vi "fourier plus standard deviation HASO.vi"(9 "starting frequency bin to plot":i32, 10 "Array in":sgl[][](array[numeric]), 11 "rep rate (Hz)":sgl) -> (1 "Power spectral density":cluster{"f0":dbl, "df":dbl, "magnitude":dbl[]}[](array[cluster]), 2 "Sds":dbl[](array[numeric]), 3 "Power spectra":cluster{"f0":dbl, "df":dbl, "magnitude":dbl[]}[](array[cluster]))   [LabVIEW 2020]
uses:
  <vilib>/Analysis/NI_AALBase.lvlib
panel:
  out "x/y":dbl[](array[numeric])
  out "delta t":sgl
  out "Num points":i32
  out "SDs from Power spectral density":dbl[](array[numeric])
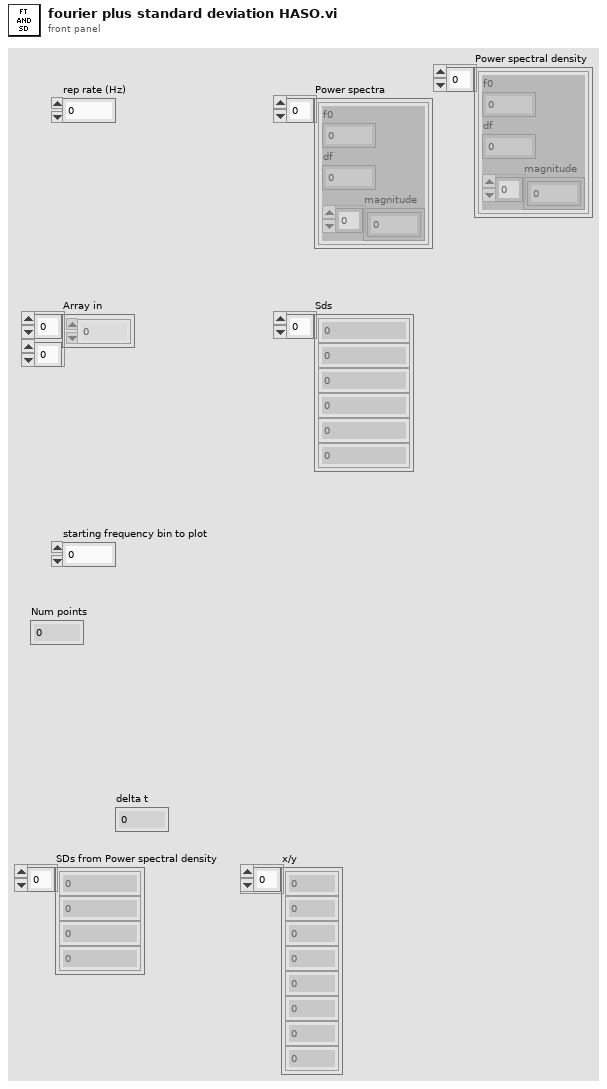
[diagram p1: front panel]
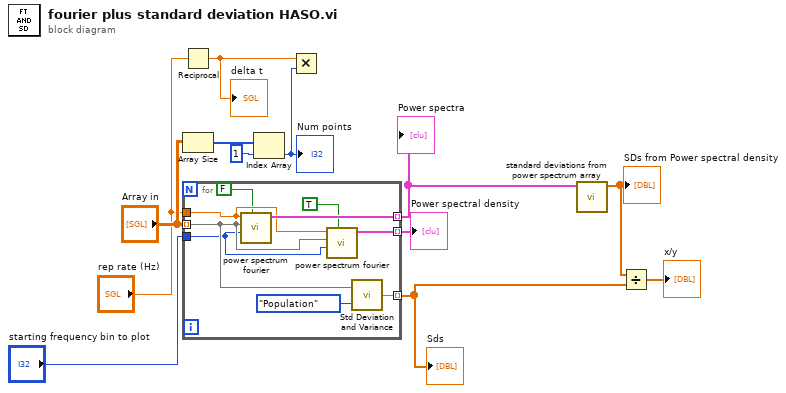
[diagram p0: block diagram]
diagram:
  n1 = Reciprocal(x="rep rate (Hz)") -> (1/x=w6:sgl)
  "delta t" <- w6
  n2 = Array Size(array="Array in") -> (size(s)=w9:i32[])
  n3 = for {
    tunnel: [w21] -> w11 mode=indexing
    tunnel: "starting frequency bin to plot" -> [w15]
    tunnel: "rep rate (Hz)" -> [w17]
    tunnel: "Array in" -> [w16] mode=indexing
    tunnel: [w20] -> w4 mode=indexing
    tunnel: [w14] -> w1 mode=indexing
    n4 = call "power spectrum fourier.vi"("PSD (T) PS (F)"=FALSE, "starting frequency bin to plot"=w15, "Array"=w16, "rep rate (Hz)"=w17) -> ("Power Spectrum"=w21:cluster{"f0":dbl, "df":dbl, "magnitude":dbl[]})  [unwired: 7 in]
    n5 = call "power spectrum fourier.vi"("PSD (T) PS (F)"=TRUE, "starting frequency bin to plot"=w15, "Array"=w16, "rep rate (Hz)"=w17) -> ("Power Spectrum"=w14:cluster{"f0":dbl, "df":dbl, "magnitude":dbl[]})  [unwired: 7 in]
    n6 = call <vilib>:"Std Deviation and Variance.vi"("X"=w16, "Weighting (Sample)"=enum16{"Sample", "Population"}."Population") -> ("standard deviation"=w20:dbl)  [unwired: 2 out]
  }
  "Sds" <- w4
  "Power spectra" <- w11
  "Power spectral density" <- w1
  n7 = Index Array(array=w9, index=1) -> (element=w5:i32)
  "Num points" <- w5
  n8 = Multiply(x=w6, y=w5) -> ()  [unwired: 1 out]
  n9 = call "standard deviations from power spectrum array.vi"("pwer spectran"=w11) -> ("standard deviations"=w2:dbl[])  [unwired: 10 in]
  "SDs from Power spectral density" <- w2
  n10 = Divide(x=w2, y=w4) -> (x/y=→"x/y":dbl[])
